vi "Sin обр.vi"() -> ()   [LabVIEW 2011]
uses:
  Control sin.ctl
panel:
  out "Waveform Chart":dbl(graph)
  in  "Numeric":dbl
  in  "stop":bool
  in  "Exit":bool
  in  "Start":bool
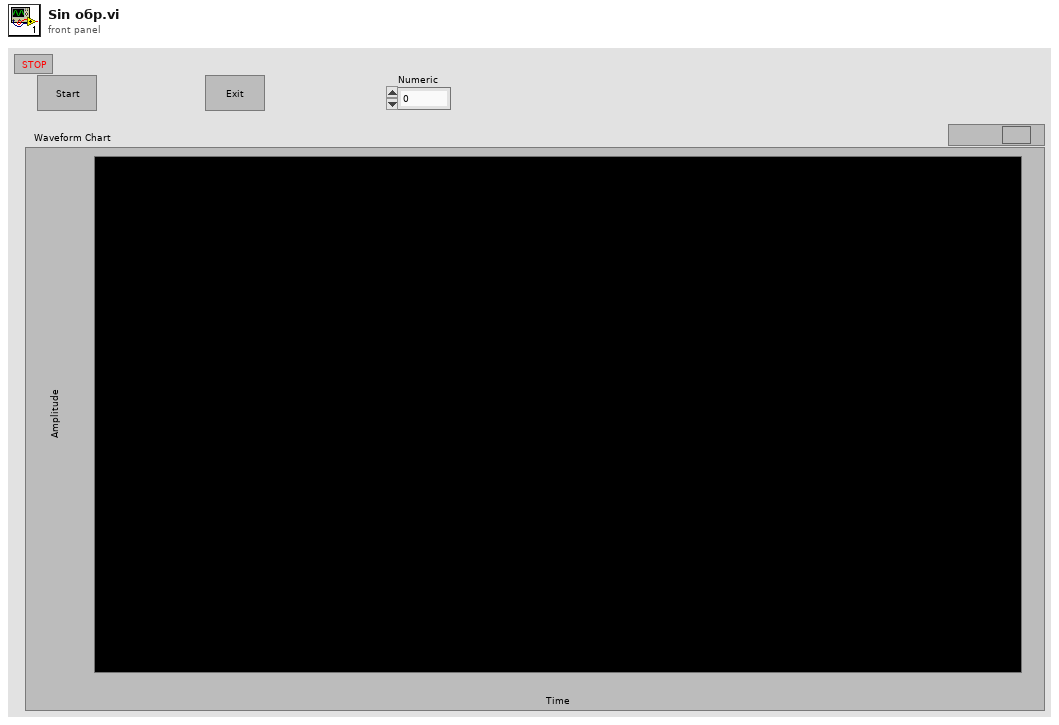
[diagram p1: front panel]
types:
  T1 = typedef "Control sin.ctl" = enum16{"Stop", "Start", "Обрізати", "Exit", "Sin"}
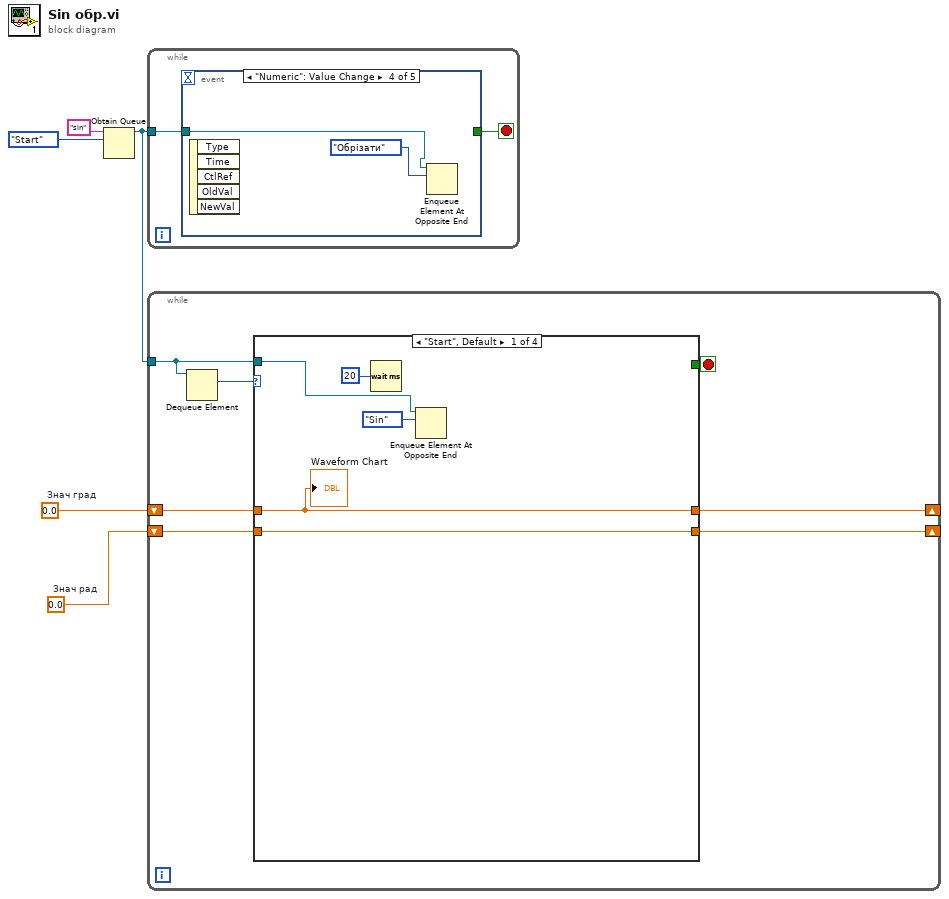
[diagram p0: block diagram]
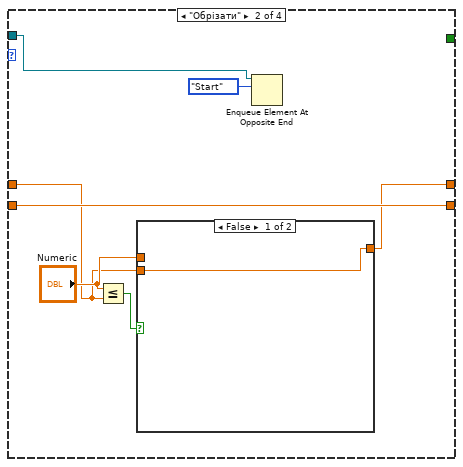
[diagram p2: hidden frame]
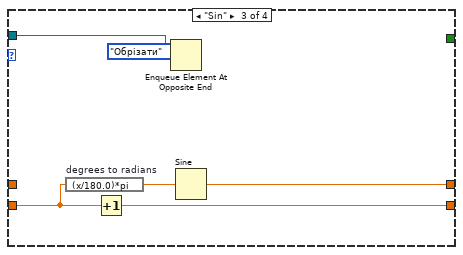
[diagram p4: hidden frame]
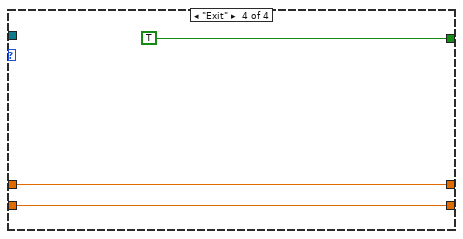
[diagram p5: hidden frame]
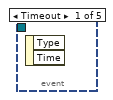
[diagram p6: hidden frame]
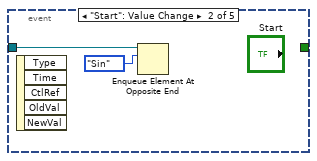
[diagram p7: hidden frame]
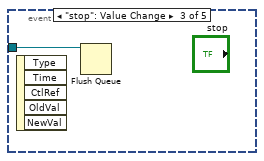
[diagram p8: hidden frame]
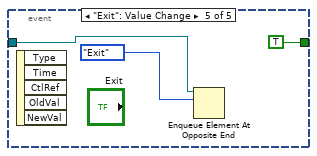
[diagram p9: hidden frame]
diagram:
  w1 = 0.0  # Знач град
  w3 = 0.0  # Знач рад
  n1 = Obtain Queue(name (unnamed)="sin", element data type=Control_sin."Start" ("Enum")) -> (queue out=w2:refnum<queue>)  [unwired: 3 in, 2 out]
  n2 = while {
    tunnel: w2 -> [w7]
    stop <- w6 stop-if-true
    n3 = event shown="[3] \"Numeric\": Value Change" {
      selector: _ -> [_ _ _ _ _]
      dyn-events: _ -> [_ _ _ _ _]
      timeout: _ -> [_ _ _ _ _]
      tunnel: w7 -> [_ w9 w10 w12 w14]
      tunnel: [_ _ _ _ TRUE] -> w6
      event Timeout {
        n4 = event-data() -> ()  [unwired: 1 in, 2 out]
      }
      event "Start": Value Change {
        n5 = event-data() -> ()  [unwired: 1 in, 5 out]
        n6 = Enqueue Element At Opposite End(queue=w9, element=Control_sin."Sin" ("Enum")) -> ()  [unwired: 2 in, 3 out]
      }
      event "stop": Value Change {
        n7 = event-data() -> ()  [unwired: 1 in, 5 out]
        n8 = Flush Queue(queue=w10) -> ()  [unwired: 1 in, 3 out]
      }
      event "Numeric": Value Change {
        n9 = event-data() -> ()  [unwired: 1 in, 5 out]
        n10 = Enqueue Element At Opposite End(queue=w12, element=Control_sin."Обрізати" ("Enum")) -> ()  [unwired: 2 in, 3 out]
      }
      event "Exit": Value Change {
        n11 = event-data() -> ()  [unwired: 1 in, 5 out]
        n12 = Enqueue Element At Opposite End(queue=w14, element=Control_sin."Exit" ("Enum")) -> ()  [unwired: 2 in, 3 out]
      }
    }
  }
  n13 = while {
    tunnel: w2 -> [w16]
    shift-right: [w19] -> _
    shift-left: w3 -> [w21]
    shift-right: [w18] -> _
    shift-left: w1 -> [w17]
    stop <- w20 stop-if-true
    n14 = Dequeue Element(queue=w16) -> (element=w22:T1)  [unwired: 2 in, 3 out]
    n15 = case shown="\"Start\", Default" w22 {
      tunnel: w21 -> [w27 w31 w41 w45]
      tunnel: [w27 w31 w40 w45] -> w19
      tunnel: [_ _ _ TRUE] -> w20
      tunnel: [w23 w30 w39 w43] -> w18
      tunnel: w17 -> [w23 w28 _ w43]
      tunnel: w16 -> [w25 w32 w37 _]
      frame "Start", Default {
        n16 = Wait (ms)(milliseconds to wait=u32 20) -> ()  [unwired: 1 out]
        n17 = Enqueue Element At Opposite End(queue=w25, element=Control_sin."Sin" ("Enum")) -> ()  [unwired: 2 in, 3 out]
        "Waveform Chart" <- w23
      }
      frame "Обрізати" {
        n18 = Less Or Equal?(x="Numeric", y=w28) -> (x <= y?=w34:bool)
        n19 = case shown="False" w34 {
          tunnel: "Numeric" -> [_ w36]
          tunnel: [w35 w36] -> w30
          tunnel: w28 -> [w35 _]
          frame False {
          }
          frame True {
          }
        }
        n20 = Enqueue Element At Opposite End(queue=w32, element=Control_sin."Start" ("Enum")) -> ()  [unwired: 2 in, 3 out]
      }
      frame "Sin" {
        n21 = expression code="(x/180.0)*pi" "degrees to radians"(w41) -> (w42:dbl)
        n22 = Increment(x=w41) -> (x+1=w40:dbl)
        n23 = Enqueue Element At Opposite End(queue=w37, element=Control_sin."Обрізати" ("Enum")) -> ()  [unwired: 2 in, 3 out]
        n24 = Sine(x=w42) -> (sin(x)=w39:dbl)
      }
      frame "Exit" {
      }
    }
  }
